vi "Traffic Light Controller (Red).vi"(7 "peds stopped":T1) -> (0 "traffic light":T2, 3 "cars stopped":T1)   [LabVIEW 2023]
uses:
  <extravilib>/ChannelInstances/One Element Stream-u16/)Channel.ctl
  <extravilib>/ChannelInstances/One Element Stream-bool/)Channel.ctl
  0d493caf-0f13-4f40-9c9a-86f422a7d2f1.vi
  04fc8c90-0391-3c46-9268-aa9e1964be30.vi
  <extravilib>/ChannelInstances/One Element Stream-u16/Write With Abort.vi
  <extravilib>/ChannelInstances/One Element Stream-bool/Write With Abort.vi
  <extravilib>/ChannelInstances/One Element Stream-bool/Read With Abort.vi
  <extravilib>/ChannelInstances/One Element Stream-u16/Endpoint.vi
  <extravilib>/ChannelInstances/One Element Stream-bool/Endpoint.vi
  <extravilib>/ChannelInstances/One Element Stream-bool/EndpointRead.vi
  <extravilib>/ChannelInstances/One Element Stream-bool.lvlib
  <extravilib>/ChannelInstances/One Element Stream-u16.lvlib
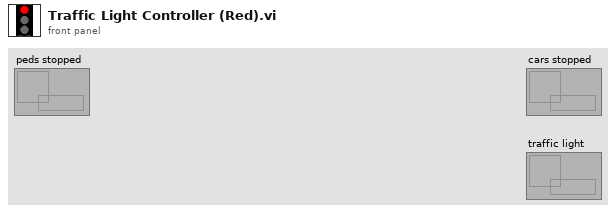
[diagram p1: front panel]
types:
  T1 = typedef "One Element Stream-bool.lvlib/)Channel.ctl" = refnum<queue>
  T2 = typedef "One Element Stream-u16.lvlib/)Channel.ctl" = refnum<queue>
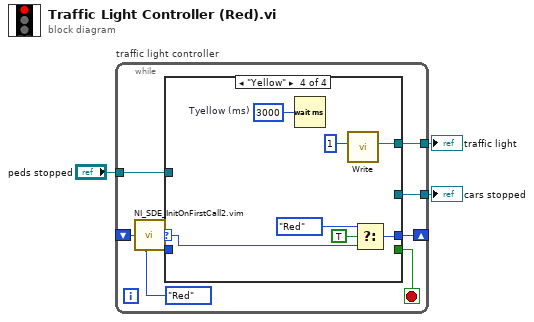
[diagram p0: block diagram]
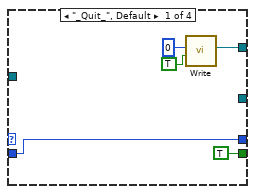
[diagram p2: hidden frame]
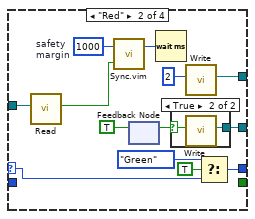
[diagram p3: hidden frame]
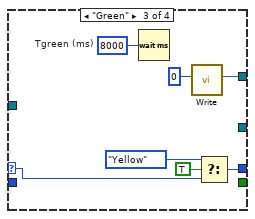
[diagram p5: hidden frame]
diagram:
  n1 = while "traffic light controller" {
    tunnel: "peds stopped" -> [w10]
    tunnel: [w9] -> w3
    tunnel: [w8] -> w2
    shift-right: [w6] -> _
    shift-left: _ -> [w5]
    stop <- w11 stop-if-true
    w7 = enum16{"_Quit_", "Red", "Green", "Yellow"}."Red"
    n2 = call "NI_SDE_InitOnFirstCall2.vim"("input"=w5, "master enum"=w7) -> ("output enum"=w4:enum16{"_Quit_", "Red", "Green", "Yellow"})  [unwired: 1 in]
    n3 = case shown="\"Yellow\"" w4 {
      selector: w4 -> [_ w29 w38 w45]
      tunnel: [TRUE _ _ _] -> w11
      tunnel: [w12 w28 w37 w44] -> w6
      tunnel: w10 -> [_ w26 _ _]
      tunnel: [w14 w24 w32 w42] -> w9
      tunnel: [_ w23 _ _] -> w8
      tunnel: w7 -> [w12 _ _ _]
      frame "_Quit_", Default {
        n4 = call <extravilib>:"Write.vi"("last element? (F)"=TRUE, "element"=u16 0) -> ("channel"=w14:T2)  [unwired: 8 in, 1 out]
      }
      frame "Red" {
        w20 = u32 1000  # safety margin
        n5 = call <extravilib>:"Read.vi"("channel"=w26) -> ("element"=w21:bool)  [unwired: 7 in, 3 out]
        n6 = call "Sync.vim"("a"=w20, "b"=w21) -> ("a'"=w19:u32)  [unwired: 24 in, 1 out]
        n7 = feedback-in #1(TRUE) -> ()
        n8 = feedback #1() -> (w17:bool)  [unwired: 1 in]
        n9 = Wait (ms)(milliseconds to wait=w19) -> ()  [unwired: 1 out]
        n10 = case shown="True" w17 {
          selector: w17 -> [_ w30]
          tunnel: [_ w31] -> w23
          frame False {
          }
          frame True {
            n11 = call <extravilib>:"Write.vi"("element"=w30) -> ("channel"=w31:T1)  [unwired: 9 in, 1 out]
          }
        }
        n12 = call <extravilib>:"Write.vi"("element"=u16 2) -> ("channel"=w24:T2)  [unwired: 9 in, 1 out]
        n13 = Select(t=enum16{"_Quit_", "Red", "Green", "Yellow"}."Green", s=TRUE, f=w29) -> (s? t:f=w28:enum16{"_Quit_", "Red", "Green", "Yellow"})
      }
      frame "Green" {
        w35 = u32 8000  # Tgreen (ms)
        n14 = Wait (ms)(milliseconds to wait=w35) -> ()  [unwired: 1 out]
        n15 = call <extravilib>:"Write.vi"("element"=u16 0) -> ("channel"=w32:T2)  [unwired: 9 in, 1 out]
        n16 = Select(t=enum16{"_Quit_", "Red", "Green", "Yellow"}."Yellow", s=TRUE, f=w38) -> (s? t:f=w37:enum16{"_Quit_", "Red", "Green", "Yellow"})
      }
      frame "Yellow" {
        w39 = u32 3000  # Tyellow (ms)
        n17 = Wait (ms)(milliseconds to wait=w39) -> ()  [unwired: 1 out]
        n18 = call <extravilib>:"Write.vi"("element"=u16 1) -> ("channel"=w42:T2)  [unwired: 9 in, 1 out]
        n19 = Select(t=enum16{"_Quit_", "Red", "Green", "Yellow"}."Red", s=TRUE, f=w45) -> (s? t:f=w44:enum16{"_Quit_", "Red", "Green", "Yellow"})
      }
    }
  }
  "traffic light" <- w3
  "cars stopped" <- w2
